vi "GenerateExpectedWaveformgraphusingLabVIEW.vi"() -> (0 "error out":errorcluster)   [LabVIEW 2010]
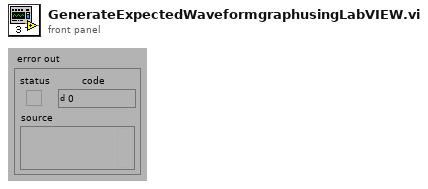
[diagram p1: front panel]
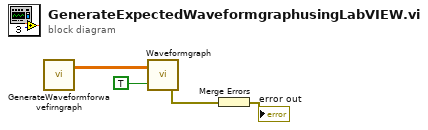
[diagram p0: block diagram]
diagram:
  n1 = call "GenerateWaveformforwavefirngraph.vi"() -> ("Waveform Graph"=w1:dbl[][])  [unwired: 3 out]
  n2 = call "Waveformgraph.vi"("Save Current Image"=TRUE, "Waveform Graph"=w1) -> ("error out"=w3:errorcluster)  [unwired: 1 out]
  n3 = Merge Errors(w3) -> (→"error out":errorcluster)
